vi "Get configuration chain.vi"(8 "error in (no error)":errorcluster, 11 "LineCCDBase in":refnum<class "LineCCD.lvclass">) -> (0 "error out":errorcluster, 1 "class name":string[](array[string]), 2 "configuration chain":variant[](array[variant]), 3 "LineCCDBase out":refnum<class "LineCCD.lvclass">)   [LabVIEW 2012, in "LineCCD.lvclass"]
doc: "Returns an array of variants containing the configuration clusters of each class in the inheritance chain (lowest child class first), together with an array of all class names in the inheritance chain.\n\nFor classes without configuration cluster, the configuration chain contains empty variants."
uses:
  LineCCD.lvclass
  <vilib>/Distrio/Murmex/Murmex/Murmex.lvclass
  LineCCD.lvclass/LineCCD.ctl
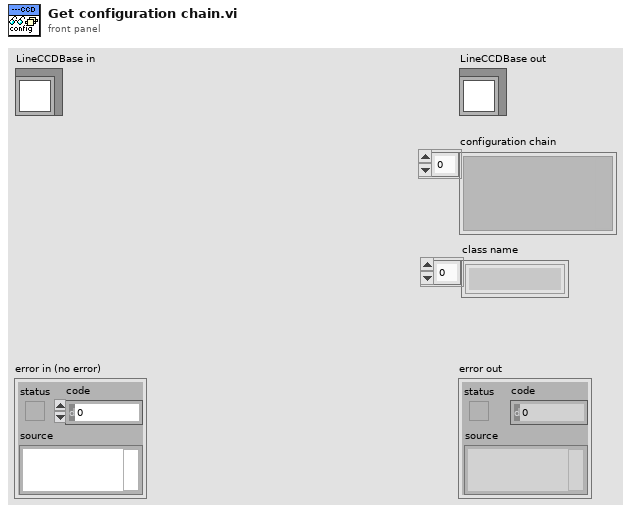
[diagram p1: front panel]
types:
  T1 = typedef "LineCCD.lvclass/configuration.ctl" = cluster{"Numeric":dbl}
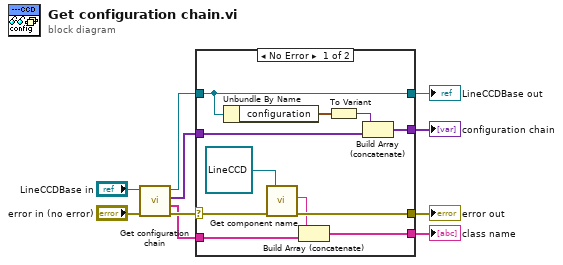
[diagram p0: block diagram]
diagram:
  n1 = call-parent "Get configuration chain.vi"("error in (no error)"="error in (no error)", "MurmexBase in"="LineCCDBase in") -> ("error out"=w8:errorcluster, "class name"=w4:string[], "configuration chain"=w6:variant[], "MurmexBase out"=w7:refnum<class "LineCCD.lvclass">)  [unwired: 6 in]
  n2 = case shown="No Error" w8 {
    selector: w8 -> [w18 w23]
    tunnel: w7 -> [w12 w25]
    tunnel: w6 -> [w19 w24]
    tunnel: [w16 w23] -> w5
    tunnel: w4 -> [w14 w22]
    tunnel: [w13 w22] -> w3
    tunnel: [w12 w25] -> w2
    tunnel: [w11 w24] -> w1
    frame No Error {
      n3 = Unbundle By Name(w12) -> ("configuration"=w20:T1)
      n4 = call <vilib>:"Get component name.vi"("error in (no error)"=w18, "Murmex in"=refnum<class "LineCCD.lvclass"> refnum ("LineCCD.lvclass")) -> ("error out"=w16:errorcluster, "component name"=w15:string)  [unwired: 7 in, 1 out]
      n5 = Build Array (concatenate)(w15, w14) -> (w13:string[])
      n6 = To Variant(anything=w20) -> (Variant=w21:variant)
      n7 = Build Array (concatenate)(w21, w19) -> (w11:variant[])
    }
    frame Error {
    }
  }
  "error out" <- w5
  "LineCCDBase out" <- w2
  "configuration chain" <- w1
  "class name" <- w3
